vi "Validate Configuration.vi"(8 "error in":errorcluster, 11 "IValidateConfiguration in":refnum<class "IValidate Configuration.lvclass">) -> (0 "error out":errorcluster, 3 "IValidateConfiguration out":refnum<class "IValidate Configuration.lvclass">)   [LabVIEW 2025, in "IValidate Configuration.lvclass"]
uses:
  IValidate Configuration.lvclass
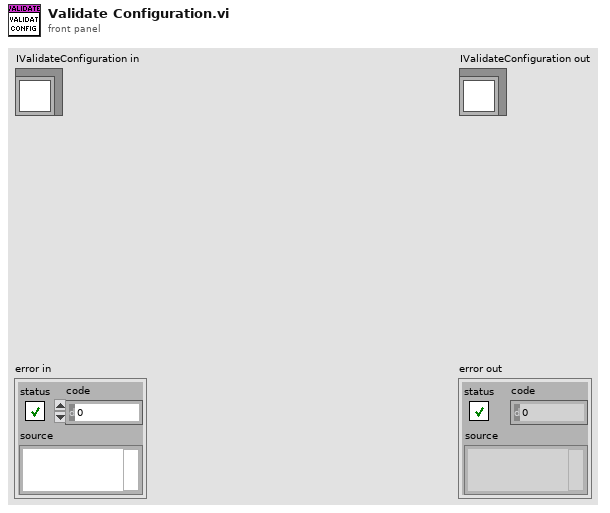
[diagram p1: front panel]
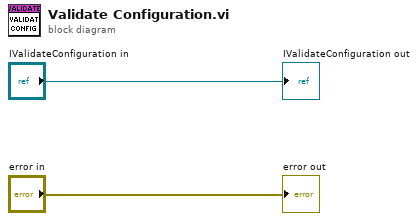
[diagram p0: block diagram]
diagram:
  "error out" <- "error in"
  "IValidateConfiguration out" <- "IValidateConfiguration in"
